vi "Main.vi"() -> ()   [LabVIEW 2015]
uses:
  TypeDefs/Buttons UI.ctl
  TypeDefs/States.ctl
  TypeDefs/Acq Loop Data.ctl
panel:
  in  "#samples":dbl=100.0
  in  "Frequency":dbl=1000.0
  out "File Path":path
  in  "File Name Prefix":string="LV Academy"
  in  "Buttons":T1
  out "Wykres":dbl[](graph)
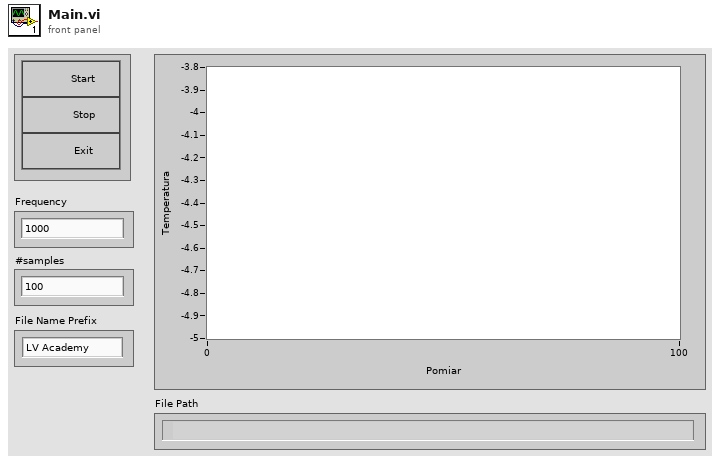
[diagram p1: front panel]
types:
  T1 = typedef "Buttons UI.ctl" = cluster{"Start":bool, "Stop":bool, "Exit":bool}
  T2 = typedef "Acq Loop Data.ctl" = cluster{"File Name Profix":string, "Frequency":dbl, "#samples":i32, "DAQ task ":refnum<k21>}
  T3 = typedef "Queue Data" = cluster{"Action":string, "Data":dbl[], "kana³":string}
  T4 = typedef "States.ctl" = enum16{"Check if Stop or Exit", "Exit", "Wait for Start or Exit", "Start Acquisition", "Reset Acquisition", "Acquisition"}
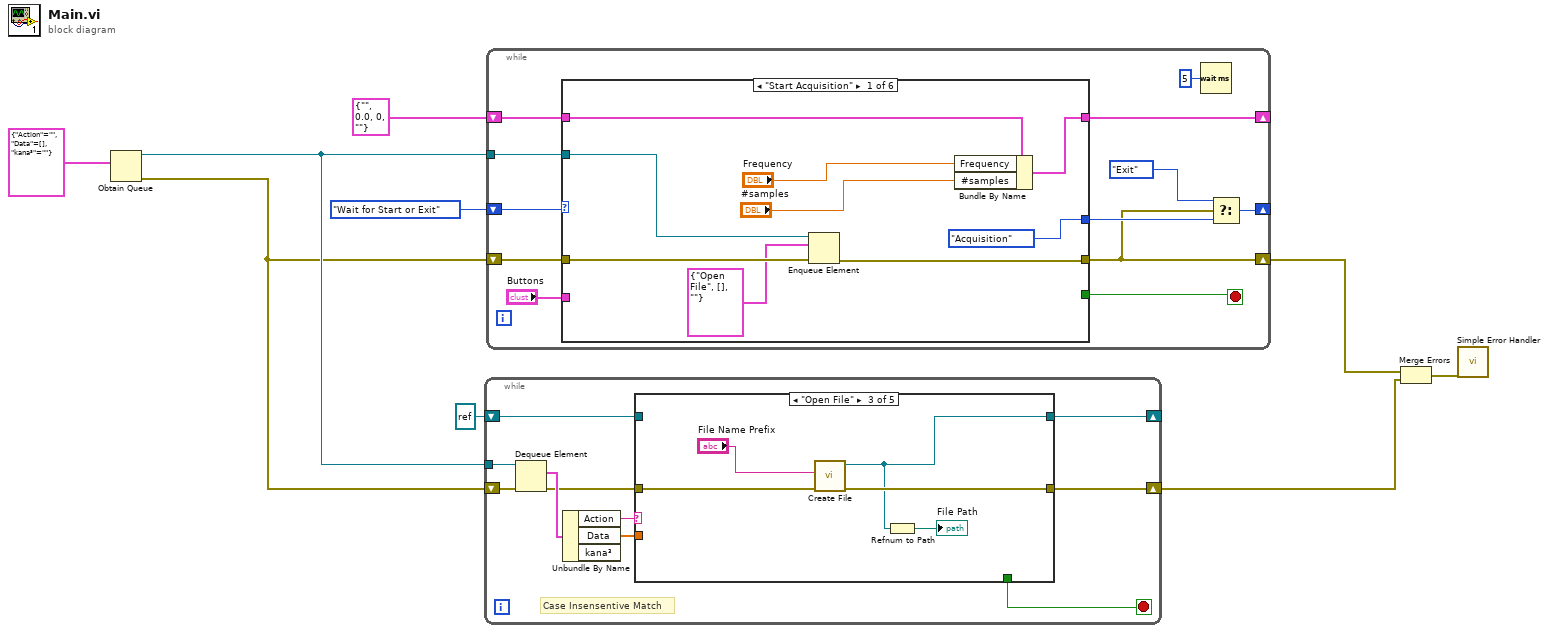
[diagram p0: block diagram]
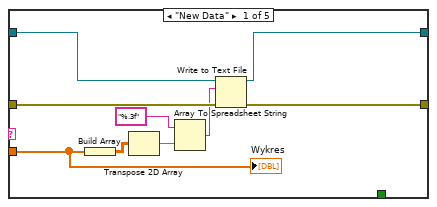
[diagram p2: hidden frame]
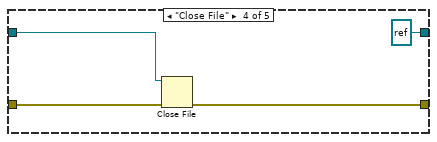
[diagram p4: hidden frame]
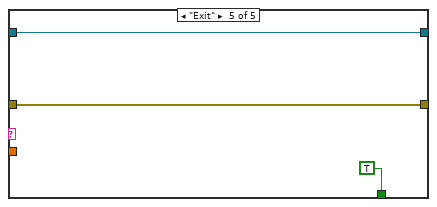
[diagram p5: hidden frame]
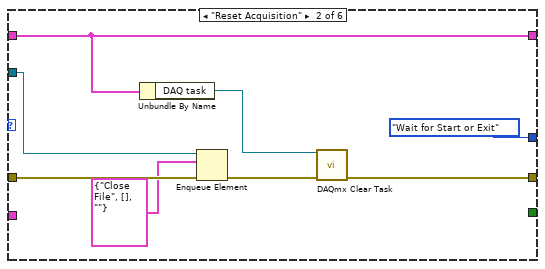
[diagram p6: hidden frame]
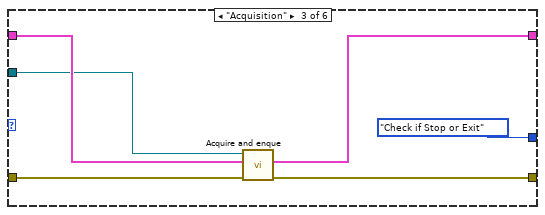
[diagram p7: hidden frame]
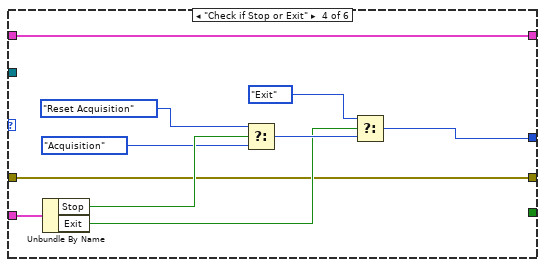
[diagram p8: hidden frame]
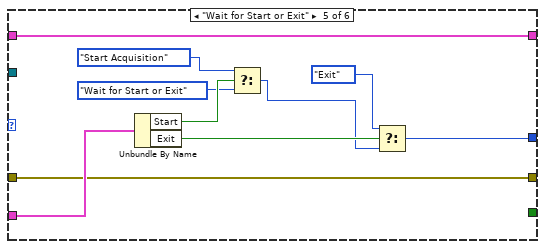
[diagram p9: hidden frame]
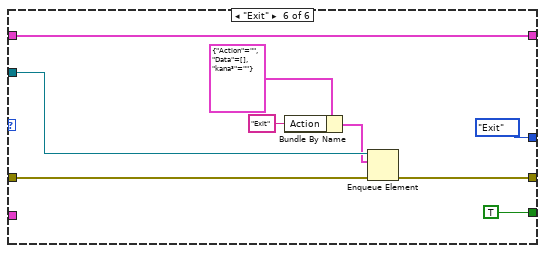
[diagram p10: hidden frame]
diagram:
  n1 = Obtain Queue(element data type=T3 {"Action"="", "Data"=[], "kana³"=""}) -> (queue out=w7:refnum<queue>, error out=w6:errorcluster)  [unwired: 4 in, 1 out]
  n2 = while {
    tunnel: w7 -> [w19]
    shift-right: [w12] -> w3
    shift-left: w6 -> [w18]
    shift-right: [w13] -> _
    shift-left: refnum<file> refnum ("refnum out") -> [w11]
    stop <- w10 stop-if-true
    # "Case Insensentive Match"
    n3 = Dequeue Element(queue=w19, error in (no error)=w18) -> (element=w17:T3, error out=w14:errorcluster)  [unwired: 1 in, 2 out]
    n4 = Unbundle By Name(w17) -> ("Action"=w16:string, "Data"=w15:dbl[])  [unwired: 1 out]
    n5 = case shown="\"Open File\"" w16 {
      tunnel: w15 -> [w22 _ _ _ _]
      tunnel: w14 -> [w27 w30 w35 w39 w41]
      tunnel: [w24 w29 w31 refnum<file> refnum ("refnum out") w40] -> w13
      tunnel: [w23 w30 w33 w37 w41] -> w12
      tunnel: w11 -> [w25 w29 _ w38 w40]
      tunnel: [_ _ _ _ TRUE] -> w10
      frame "New Data" {
        n6 = Build Array(w22) -> (w20:dbl[][])
        n7 = Transpose 2D Array(2D array=w20) -> (transposed array=w21:dbl[][])
        n8 = Array To Spreadsheet String(array=w21, 3:"%.3f") -> (spreadsheet string=w26:string)  [unwired: 1 in]
        n9 = Write to Text File(file (use dialog)=w25, text=w26, error in=w27) -> (refnum out=w24:refnum<file>, error out=w23:errorcluster)  [unwired: 1 in, 1 out]
        "Wykres" <- w22
      }
      frame Default {
      }
      frame "Open File" {
        n10 = call "Create File.vi"("error in (no error)"=w35, "File Name Prefix"="File Name Prefix") -> ("error out"=w33:errorcluster, "refnum out"=w31:refnum<file>)  [unwired: 8 in]
        n11 = Refnum to Path(1:w31) -> (0:→"File Path":path)
      }
      frame "Close File" {
        n12 = Close File(refnum=w38, error in=w39) -> (error out=w37:errorcluster)  [unwired: 1 out]
      }
      frame "Exit" {
      }
    }
  }
  n13 = while {
    shift-right: [w45] -> _
    shift-left: States."Wait for Start or Exit" -> [w54]
    tunnel: w7 -> [w52]
    shift-right: [w49] -> _
    shift-left: T2 {"File Name Profix"="", "Frequency"=0.0, "#samples"=0, "DAQ task "=""} -> [w50]
    shift-right: [w43] -> w2
    shift-left: w6 -> [w53]
    stop <- w47 stop-if-true
    n14 = case shown="\"Start Acquisition\"" w54 {
      tunnel: w53 -> [w58 w68 w77 w79 w90 w105]
      tunnel: w52 -> [w56 w66 w75 _ _ w103]
      tunnel: "Buttons" -> [_ _ _ w87 w97 _]
      tunnel: [States."Acquisition" States."Wait for Start or Exit" States."Check if Stop or Exit" w80 w92 States."Exit"] -> w46
      tunnel: w50 -> [w63 w64 w76 w78 w91 w99]
      tunnel: [w60 w64 w72 w78 w91 w99] -> w49
      tunnel: [w57 w71 w74 w79 w90 w104] -> w43
      tunnel: [_ _ _ _ _ TRUE] -> w47
      frame "Start Acquisition" {
        n15 = Enqueue Element(queue=w56, element=T3 {"Action"="Open File", "Data"=[], "kana³"=""}, error in (no error)=w58) -> (error out=w57:errorcluster)  [unwired: 1 in, 2 out]
        n16 = Bundle By Name(cluster=w63, "Frequency"="Frequency", "#samples"="#samples") -> (w60:T2)
      }
      frame "Reset Acquisition" {
        n17 = Unbundle By Name(w64) -> ("DAQ task"=w70:refnum<k21>)
        n18 = Enqueue Element(queue=w66, element=T3 {"Action"="Close File", "Data"=[], "kana³"=""}, error in (no error)=w68) -> (error out=w67:errorcluster)  [unwired: 1 in, 2 out]
        n19 = call <vilib>:"DAQmx Clear Task.vi"("task in"=w70, "error in"=w67) -> ("error out"=w71:errorcluster)  [unwired: 13 in]
      }
      frame "Acquisition" {
        n20 = call "Acquire and enque.vi"("error in (no error)"=w77, "Data In"=w76, "Queue in"=w75) -> ("error out"=w74:errorcluster, "Data Out"=w72:T2)  [unwired: 7 in]
      }
      frame "Check if Stop or Exit" {
        n21 = Unbundle By Name(w87) -> ("Stop"=w86:bool, "Exit"=w82:bool)
        n22 = Select(t=States."Reset Acquisition", s=w86, f=States."Acquisition") -> (s? t:f=w83:T4)
        n23 = Select(t=States."Exit", s=w82, f=w83) -> (s? t:f=w80:T4)
      }
      frame "Wait for Start or Exit" {
        n24 = Unbundle By Name(w97) -> ("Start"=w96:bool, "Exit"=w93:bool)
        n25 = Select(t=States."Start Acquisition", s=w96, f=States."Wait for Start or Exit") -> (s? t:f=w89:T4)
        n26 = Select(t=States."Exit", s=w93, f=w89) -> (s? t:f=w92:T4)
      }
      frame "Exit" {
        n27 = Bundle By Name(cluster=T3 {"Action"="", "Data"=[], "kana³"=""}, "Action"="Exit") -> (w100:T3)
        n28 = Enqueue Element(queue=w103, element=w100, error in (no error)=w105) -> (error out=w104:errorcluster)  [unwired: 1 in, 2 out]
      }
    }
    n29 = Wait (ms)(milliseconds to wait=u32 5) -> ()  [unwired: 1 out]
    n30 = Select(t=States."Exit", s=w43, f=w46) -> (s? t:f=w45:T4)
  }
  n31 = Merge Errors(w2, w3) -> (w1:errorcluster)
  n32 = call <vilib>:"Simple Error Handler.vi"("error in (no error)"=w1) -> ()  [unwired: 4 in, 5 out]
